vi "Delete Convolution 32f.vi"(8 "Error In":errorcluster, 11 "Convolution Object":T1 {"Convolved Memory Object"."Dimension"."Width" min=1; "Convolved Memory Object"."Dimension"."Height" min=1; "Convolved Memory Object"."Dimension"."Depth" min=1; "Kernel Memory Object"."Dimension"."Width" min=1; "Kernel Memory Object"."Dimension"."Height" min=1; "Kernel Memory Object"."Dimension"."Depth" min=1}) -> (0 "Error Out":errorcluster)   [LabVIEW 2012, in "OpenCLV x64.lvlib"]
doc: "Deletes the Kernel Memory Object, Convolution Memory Object, and deletes the convolution program."
uses:
  OpenCLV x64.lvlib
  Controls/Convolution Object.ctl
  Controls/Device ID.ctl
  Controls/Program Handle.ctl
  Controls/Memory Object.ctl
  Controls/Memory ID.ctl
  User Controls/Array Dimensions.ctl
  Controls/Memory Type.ctl
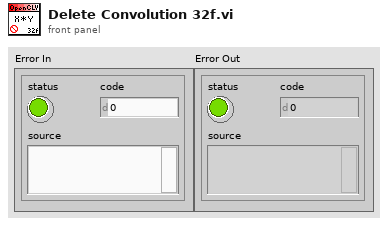
[diagram p1: front panel]
types:
  T1 = typedef "OpenCLV x64.lvlib/Convolution Object.ctl" = cluster{"Device In":T2, "Program Handle":T3, "Kernel Memory Object":T4, "Convolved Memory Object":T4}
  T2 = typedef "OpenCLV x64.lvlib/Device ID.ctl" = u64
  T3 = typedef "OpenCLV x64.lvlib/Program Handle.ctl" = u64
  T4 = typedef "OpenCLV x64.lvlib/Memory Object.ctl" = cluster{"Device ID":T2, "Memeroy ID":T5, "Dimension":T6, "Memory Type":T7}
  T5 = typedef "OpenCLV x64.lvlib/Memory ID.ctl" = u64
  T6 = typedef "Array Dimensions.ctl" = cluster{"Depth":u64, "Height":u64, "Width":u64}
  T7 = typedef "OpenCLV x64.lvlib/Memory Type.ctl" = enum16{"32f", "u8", "i8", "u16", "i16", "u32", "i32", "64f"}
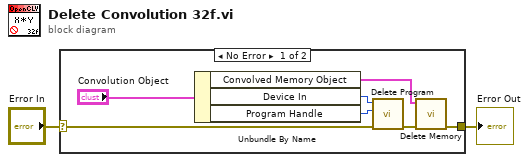
[diagram p0: block diagram]
diagram:
  n1 = case shown="No Error" "Error In" {
    selector: "Error In" -> [w7 w10]
    tunnel: [w4 w10] -> w1
    frame No Error {
      n2 = Unbundle By Name("Convolution Object") -> ("Convolved Memory Object"=w5:T4, "Device In"=w3:T2, "Program Handle"=w8:T3)
      n3 = call "Delete Program.vi"("Error In"=w7, "Program In"=w8, "Device ID"=w3) -> ("Error Out"=w6:errorcluster)  [unwired: 8 in]
      n4 = call "Delete Memory.vi"("Error In"=w6, "Memory Object In"=w5) -> ("Error Out"=w4:errorcluster)  [unwired: 8 in, 1 out]
    }
    frame Error {
    }
  }
  "Error Out" <- w1
